vi "Add Key.vi"(8 "error in (no error)":errorcluster, 9 "value":string, 10 "name":string, 11 "Topic in":refnum<class "Topic.lvclass">) -> (0 "error out":errorcluster, 2 "replaced":bool, 3 "Topic out":refnum<class "Topic.lvclass">)   [LabVIEW 2027, in "Topic.lvclass"]
uses:
  Topic.lvclass
  Topic.lvclass/Topic.ctl
  <vilib>/NI/Compiled HTML Menu Tool/Keyed Value Tree/Keyed Value Tree.lvclass
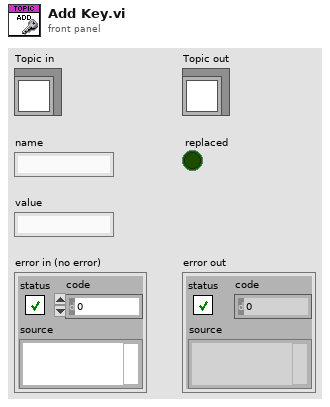
[diagram p1: front panel]
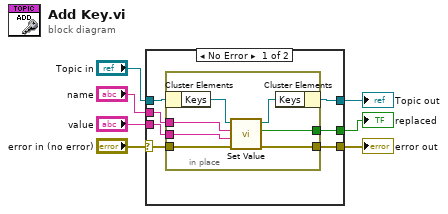
[diagram p0: block diagram]
diagram:
  n1 = case shown="No Error" "error in (no error)" {
    selector: "error in (no error)" -> [w12 w23]
    tunnel: [w11 w23] -> w6
    tunnel: [w13 w22] -> w4
    tunnel: "Topic in" -> [w14 w22]
    tunnel: [w10 _] -> w3
    tunnel: "name" -> [w9 _]
    tunnel: "value" -> [w8 _]
    frame No Error {
      n2 = in-place {
        in-place-border: w12 -> [w19]
        in-place-border: [w18] -> w11
        in-place-border: [w17] -> w10
        in-place-border: w9 -> [w16]
        in-place-border: w8 -> [w15]
        n3 = in-place-cluster #1(w14) -> ("Keys"=w21:refnum<class "Keyed Value Tree.lvclass">)
        n4 = call-dynamic "Set Value.vi"("error in (no error)"=w19, "value"=w15, "name"=w16, "Keyed Value Tree in"=w21) -> ("error out"=w18:errorcluster, "replaced"=w17:bool, "Keyed Value Tree out"=w20:refnum<class "Keyed Value Tree.lvclass">)  [unwired: 5 in]
        n5 = in-place-cluster #1("Keys"=w20) -> (w13:refnum<class "Topic.lvclass">)
      }
    }
    frame Error {
    }
  }
  "error out" <- w6
  "Topic out" <- w4
  "replaced" <- w3
